vi "ControlSystemConfiguration.vi"(0 "SV0":bool, 1 "SV1":bool, 2 "SV2":bool, 3 "SV3":bool, 4 "SV4":bool, 5 "SV5":bool, 6 "SV6":bool, 7 "Add Procedure":bool, 8 "Procedure Name":string, 9 "error in":errorcluster, 10 "P#":u32, 12 "Row":u32, 27 "Remove Procedure":bool) -> (14 "Row":u32[](array[numeric]), 16 "?":u32[](array[numeric]), 17 "error out":errorcluster[](array[cluster]), 18 "?":string[](array[string]), 19 "File Path":path[](array[path]), 20 "?":bool[](array[boolean]), 21 "?":bool[](array[boolean]), 22 "?":bool[](array[boolean]), 23 "?":bool[](array[boolean]), 24 "?":bool[](array[boolean]), 25 "?":bool[](array[boolean]), 26 "?":bool[](array[boolean]))   [LabVIEW 2021]
uses:
  <vilib>/Utility/file.llb/Write Delimited Spreadsheet (I64).vi
  <vilib>/Utility/file.llb/Write Delimited Spreadsheet (string).vi
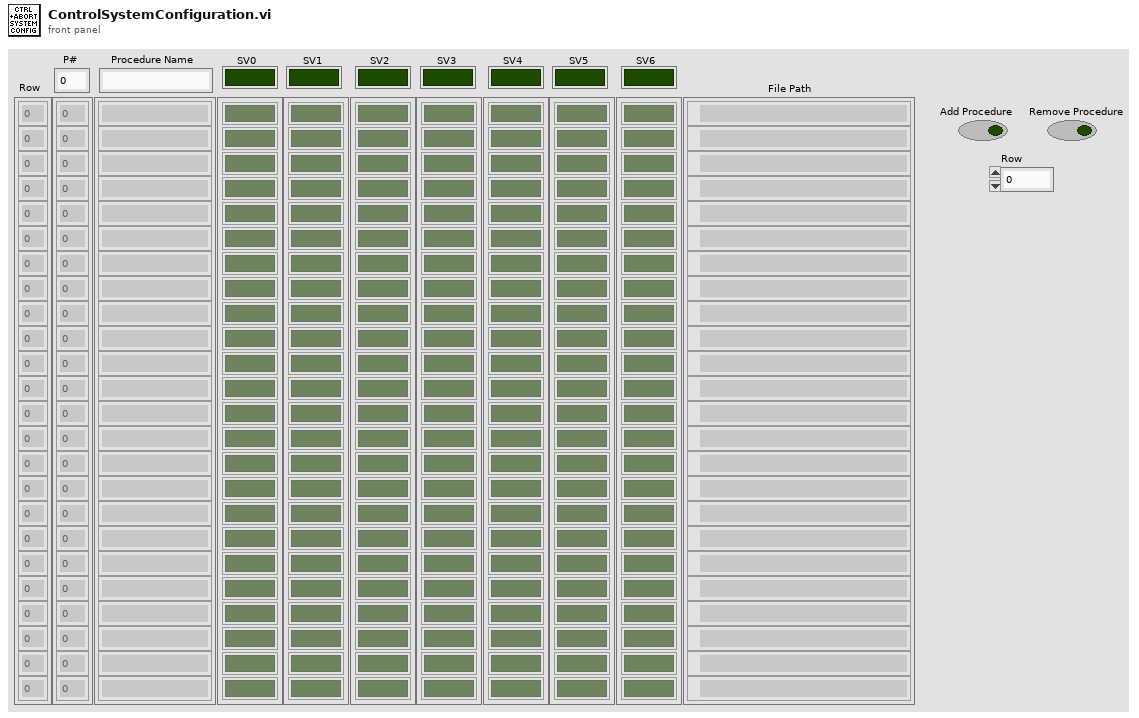
[diagram p1: front panel]
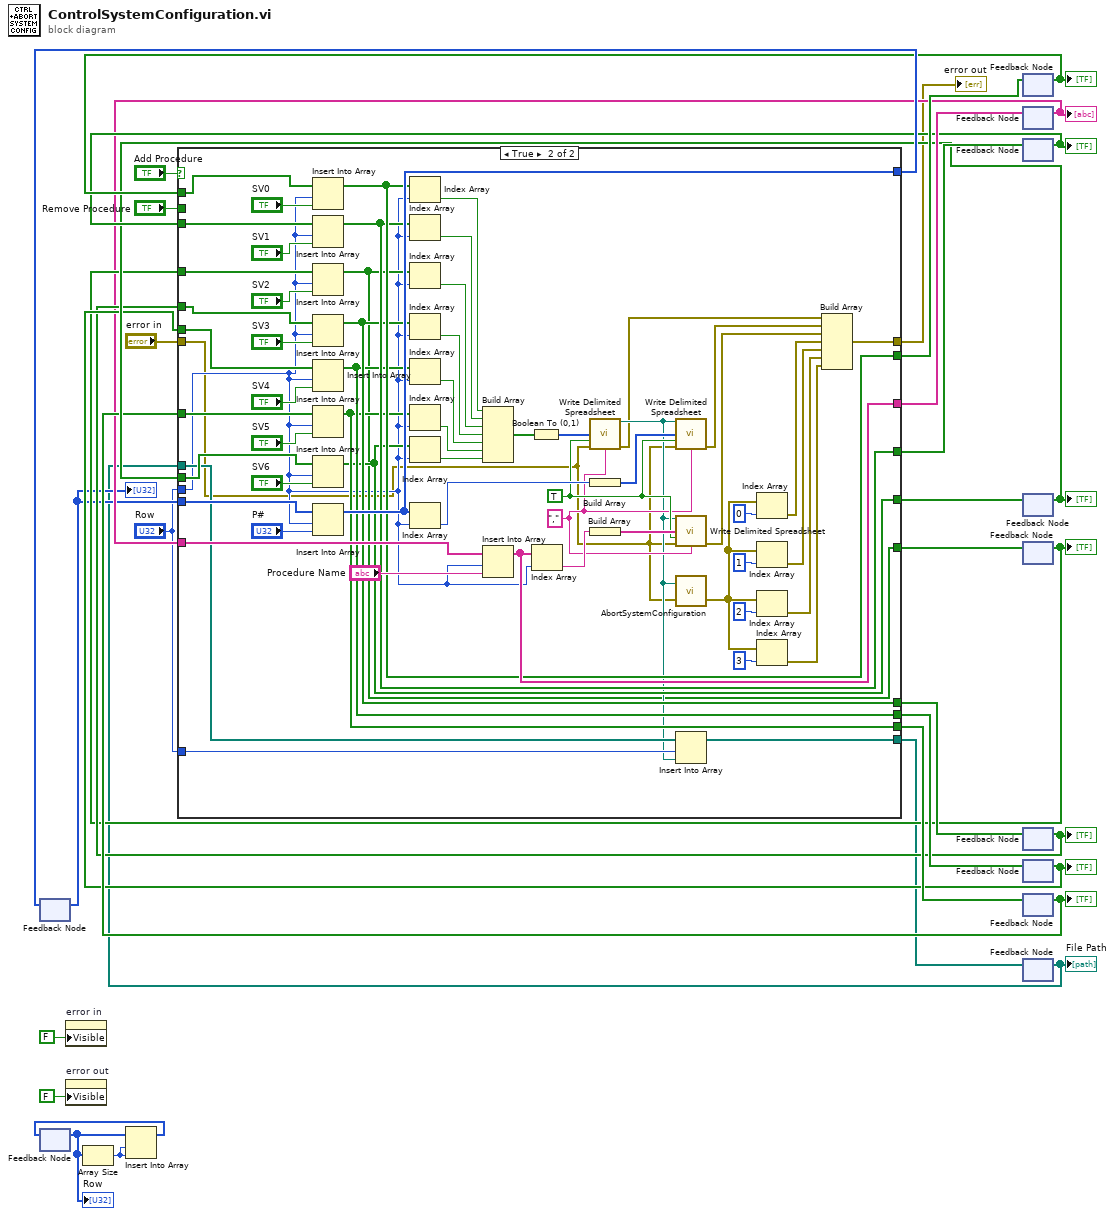
[diagram p0: block diagram]
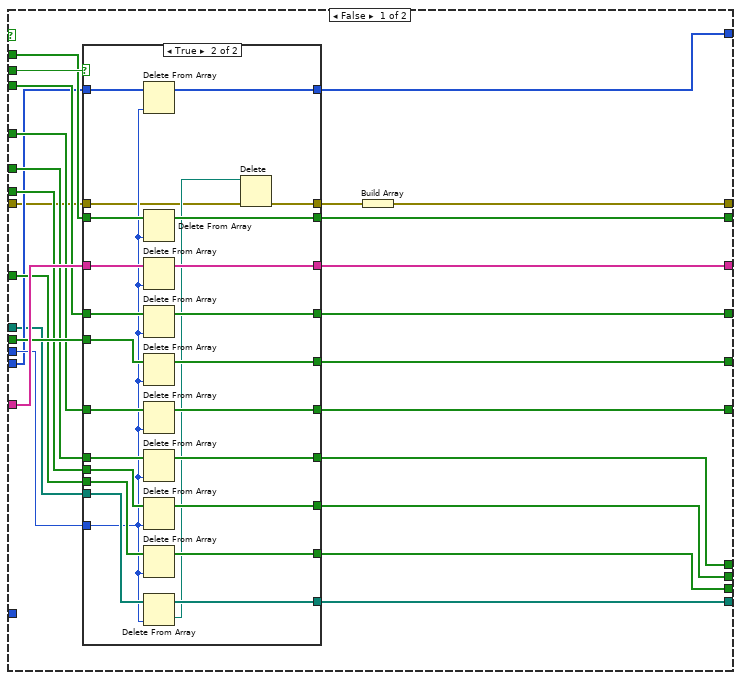
[diagram p2: hidden frame]
diagram:
  n1 = feedback #1() -> (w8:u32[])  [unwired: 1 in]
  "?" <- w8
  n2 = feedback #2() -> (w28:i32[])  [unwired: 1 in]
  "Row" <- w28
  n3 = property on="error in" class="Clust (strict)"("Visible"=FALSE) -> ()  [unwired: 2 in, 2 out]
  n4 = property on="error out" class="Arr (strict)"("Visible"=FALSE) -> ()  [unwired: 2 in, 2 out]
  n5 = Array Size(array=w28) -> (size(s)=w29:i32)
  n6 = Insert Into Array(array=w28, index=w29, new element=w29) -> (w30:i32[])
  n7 = feedback-in #2(w30) -> ()
  n8 = feedback #3() -> (w16:bool[])  [unwired: 1 in]
  "?" <- w16
  n9 = feedback #4() -> (w9:string[])  [unwired: 1 in]
  "?" <- w9
  n10 = feedback #5() -> (w15:bool[])  [unwired: 1 in]
  "?" <- w15
  n11 = feedback #6() -> (w14:bool[])  [unwired: 1 in]
  "?" <- w14
  n12 = feedback #7() -> (w10:bool[])  [unwired: 1 in]
  "?" <- w10
  n13 = feedback #8() -> (w11:bool[])  [unwired: 1 in]
  "?" <- w11
  n14 = feedback #9() -> (w12:bool[])  [unwired: 1 in]
  "?" <- w12
  n15 = feedback #10() -> (w13:bool[])  [unwired: 1 in]
  "?" <- w13
  n16 = feedback #11() -> (w5:path[])  [unwired: 1 in]
  "File Path" <- w5
  n17 = case shown="True" "Add Procedure" {
    tunnel: "Remove Procedure" -> [w55 _]
    tunnel: [w46 w116] -> w26
    tunnel: w16 -> [w47 w151]
    tunnel: w15 -> [w43 w149]
    tunnel: [w42 w115] -> w25
    tunnel: w10 -> [w45 w146]
    tunnel: [w44 w102] -> w18
    tunnel: w11 -> [w49 w144]
    tunnel: [w48 w114] -> w24
    tunnel: w12 -> [w39 w142]
    tunnel: [w38 w113] -> w23
    tunnel: w13 -> [w41 w140]
    tunnel: [w40 w112] -> w22
    tunnel: w14 -> [w51 w138]
    tunnel: [w50 w111] -> w21
    tunnel: w8 -> [w37 w136]
    tunnel: [w36 w118] -> w20
    tunnel: w9 -> [w53 w135]
    tunnel: [w54 w117] -> w19
    tunnel: "Row" -> [w52 w101]
    tunnel: "Row" -> [_ w110]
    tunnel: [w35 w109] -> w6
    tunnel: w5 -> [w34 w108]
    tunnel: "error in" -> [w33 w100]
    tunnel: [w31 w106] -> w3
    frame False {
      n18 = case shown="True" w55 {
        tunnel: [w59 w90] -> w54
        tunnel: w53 -> [w59 w89]
        tunnel: w52 -> [_ w70]
        tunnel: w51 -> [w60 w88]
        tunnel: [w60 w87] -> w50
        tunnel: w49 -> [w65 w86]
        tunnel: [w65 w85] -> w48
        tunnel: w47 -> [w63 w84]
        tunnel: [w63 w83] -> w46
        tunnel: w45 -> [w66 w82]
        tunnel: [w66 w81] -> w44
        tunnel: w43 -> [w61 w80]
        tunnel: [w61 w79] -> w42
        tunnel: w41 -> [w62 w78]
        tunnel: [w62 w77] -> w40
        tunnel: w39 -> [w64 w76]
        tunnel: [w64 w75] -> w38
        tunnel: w37 -> [w58 w73]
        tunnel: [w58 w74] -> w36
        tunnel: [w57 w72] -> w35
        tunnel: w34 -> [w57 w71]
        tunnel: w33 -> [w56 w68]
        tunnel: [w56 w67] -> w32
        frame False {
        }
        frame True {
          n19 = Delete From Array(array=w73, index=w70) -> (array with subset deleted=w74:u32[])  [unwired: 1 in, 1 out]
          n20 = Delete From Array(array=w84, index=w70) -> (array with subset deleted=w83:bool[])  [unwired: 1 in, 1 out]
          n21 = Delete From Array(array=w89, index=w70) -> (array with subset deleted=w90:string[])  [unwired: 1 in, 1 out]
          n22 = Delete From Array(array=w80, index=w70) -> (array with subset deleted=w79:bool[])  [unwired: 1 in, 1 out]
          n23 = Delete From Array(array=w88, index=w70) -> (array with subset deleted=w87:bool[])  [unwired: 1 in, 1 out]
          n24 = Delete From Array(array=w82, index=w70) -> (array with subset deleted=w81:bool[])  [unwired: 1 in, 1 out]
          n25 = Delete From Array(array=w86, index=w70) -> (array with subset deleted=w85:bool[])  [unwired: 1 in, 1 out]
          n26 = Delete From Array(array=w76, index=w70) -> (array with subset deleted=w75:bool[])  [unwired: 1 in, 1 out]
          n27 = Delete From Array(array=w78, index=w70) -> (array with subset deleted=w77:bool[])  [unwired: 1 in, 1 out]
          n28 = Delete From Array(array=w71, index=w70) -> (deleted portion=w69:path, array with subset deleted=w72:path[])  [unwired: 1 in]
          n29 = Delete(path (use dialog)=w69, error in=w68) -> (error out=w67:errorcluster)  [unwired: 3 in, 2 out]
        }
      }
      n30 = Build Array(w32) -> (w31:errorcluster[])
    }
    frame True {
      w120 = TRUE ("append to file? (new file:F)")
      w119 = "," ("delimiter (\\t)")
      n31 = Insert Into Array(array=w151, index=w101, new element="SV0") -> (w116:bool[])
      n32 = Insert Into Array(array=w149, index=w101, new element="SV1") -> (w115:bool[])
      n33 = Insert Into Array(array=w146, index=w101, new element="SV2") -> (w102:bool[])
      n34 = Insert Into Array(array=w144, index=w101, new element="SV3") -> (w114:bool[])
      n35 = Insert Into Array(array=w142, index=w101, new element="SV4") -> (w113:bool[])
      n36 = Insert Into Array(array=w140, index=w101, new element="SV5") -> (w112:bool[])
      n37 = Insert Into Array(array=w138, index=w101, new element="SV6") -> (w111:bool[])
      n38 = Insert Into Array(array=w136, index=w101, new element="P#") -> (w118:u32[])
      n39 = Index Array(array=w116, index=w101) -> (element=w130:bool)
      n40 = Index Array(array=w115, index=w101) -> (element=w127:bool)
      n41 = Index Array(array=w102, index=w101) -> (element=w128:bool)
      n42 = Index Array(array=w114, index=w101) -> (element=w133:bool)
      n43 = Index Array(array=w113, index=w101) -> (element=w129:bool)
      n44 = Index Array(array=w112, index=w101) -> (element=w132:bool)
      n45 = Index Array(array=w111, index=w101) -> (element=w131:bool)
      n46 = Index Array(array=w118, index=w101) -> (element=w122:u32)
      n47 = Build Array(w130, w127, w128, w133, w129, w132, w131) -> (w126:bool[])
      n48 = Insert Into Array(array=w135, index=w101, new element="Procedure Name") -> (w117:string[])
      n49 = Boolean To (0,1)(Boolean=w126) -> (0, 1=w125:i16[])
      n50 = Index Array(array=w117, index=w101) -> (element=w124:string)
      n51 = call-poly <vilib>:"Write Delimited Spreadsheet.vi"("1D data"=w125, "append to file? (new file:F)"=w120, "error in (no error)"=w100, "delimiter (\\t)"=w119) -> ("new file path (Not A Path if cancelled)"=w107:path, "error out"=w105:errorcluster)  [unwired: 10 in]
      n52 = Build Array(w122) -> (w121:u32[])
      n53 = Build Array(w124) -> (w123:string[])
      n54 = call-poly <vilib>:"Write Delimited Spreadsheet.vi"("file path (dialog if empty)"=w107, "1D data"=w121, "append to file? (new file:F)"=w120, "error in (no error)"=w100, "delimiter (\\t)"=w119) -> ("error out"=w104:errorcluster)  [unwired: 9 in, 1 out]
      n55 = call-poly <vilib>:"Write Delimited Spreadsheet.vi"("file path (dialog if empty)"=w107, "1D data"=w123, "append to file? (new file:F)"=w120, "error in (no error)"=w100, "delimiter (\\t)"=w119) -> ("error out"=w103:errorcluster)  [unwired: 9 in, 1 out]
      n56 = call "AbortSystemConfiguration.vi"("File Path"=w107, "error in"=w100) -> ("error out"=w95:errorcluster[])
      n57 = Insert Into Array(array=w108, index=w110, new element=w107) -> (w109:path[])
      n58 = Index Array(array=w95, index=0) -> (element=w94:errorcluster)
      n59 = Index Array(array=w95, index=1) -> (element=w93:errorcluster)
      n60 = Index Array(array=w95, index=2) -> (element=w92:errorcluster)
      n61 = Index Array(array=w95, index=3) -> (element=w91:errorcluster)
      n62 = Build Array(w105, w104, w103, w94, w93, w92, w91) -> (w106:errorcluster[])
    }
  }
  "error out" <- w3
  n63 = feedback-in #1(w20) -> ()
  n64 = feedback-in #3(w26) -> ()
  n65 = feedback-in #4(w19) -> ()
  n66 = feedback-in #5(w25) -> ()
  n67 = feedback-in #6(w21) -> ()
  n68 = feedback-in #7(w18) -> ()
  n69 = feedback-in #8(w24) -> ()
  n70 = feedback-in #9(w23) -> ()
  n71 = feedback-in #10(w22) -> ()
  n72 = feedback-in #11(w6) -> ()
